vi "Get Method Output Message.vi"(8 "error in (no error)":errorcluster, 11 "Method ref in":u64) -> (0 "error out":errorcluster, 2 "Message ref out":u64, 3 "Method ref out":u64)   [LabVIEW 2019, in "gRPC Scripting Tools.lvlib"]
uses:
  gRPC Scripting Tools.lvlib
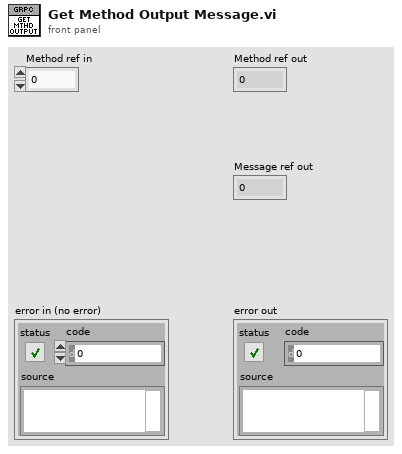
[diagram p1: front panel]
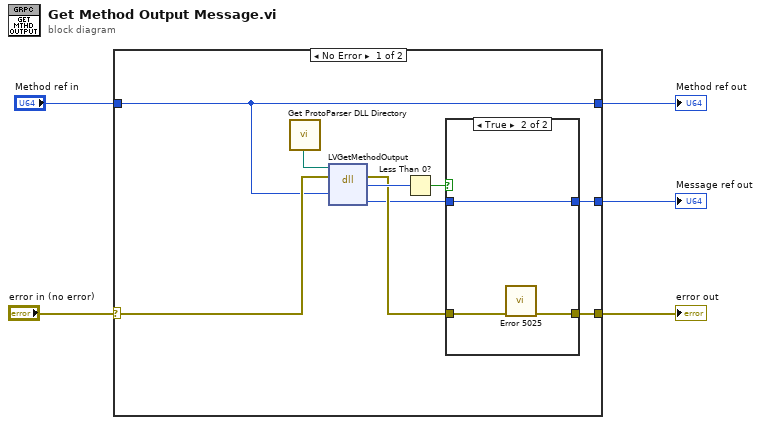
[diagram p0: block diagram]
diagram:
  n1 = case shown="No Error" "error in (no error)" {
    selector: "error in (no error)" -> [w13 w21]
    tunnel: "Method ref in" -> [w12 w20]
    tunnel: [w6 _] -> w4
    tunnel: [w12 w20] -> w2
    tunnel: [w8 w21] -> w1
    frame No Error {
      n2 = call "Get ProtoParser DLL Directory.vi"() -> ("Proto Parser Directory"=w14:path)
      n3 = dll-call lib="C:/Users/XEnderMD/Desktop/LV gRPC/labview source/gRPC Scripting Tools/Proto Parser API/dll/labview_grpc_generator.dll" fn="LVGetMethodOutput"(path in=w14, error in=w13, "method"=w12) -> (error out=w9:errorcluster, "return type"=w11:i32, "methodOutput"=w7:u64)  [unwired: 3 in, 1 out]
      n4 = Less Than 0?(x=w11) -> (x < 0?=w10:bool)
      n5 = case shown="True" w10 {
        tunnel: w9 -> [w16 w19]
        tunnel: [w16 w18] -> w8
        tunnel: w7 -> [w15 w17]
        tunnel: [w15 w17] -> w6
        frame False {
        }
        frame True {
          n6 = call "Error 5025.vi"("error in (no error)"=w19) -> ("error out"=w18:errorcluster)  [unwired: 10 in]
        }
      }
    }
    frame Error {
    }
  }
  "Message ref out" <- w4
  "Method ref out" <- w2
  "error out" <- w1
